vi "S2C_UNITHERM_Proc_Globals.vi"() -> ()   [LabVIEW 2024]
panel:
  out "Uni-Errors":cluster{"Code":i32, "Source":string}[](array[cluster])=[{"Code"=6000, "Source"="A error occurred while attempting to send an event-level local command."}, {"Code"=6001, "Source"="A error occurred while attempting to clear the communications log."}]
  in  "Uni-Visa":refnum<visa-resource-name>
  out "Uni-Refs":string[][](array[string])
  in  "Uni-VI":refnum<vi>
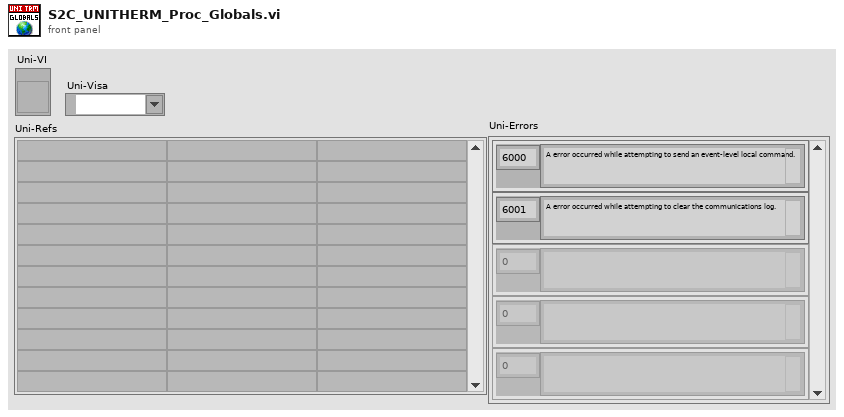
[diagram p1: front panel]
diagram:
